vi "InitDeviceAD_8532.vi"(7 "error in (no error)":errorcluster, 10 "task":T1={"Task Info"={"Accele Task"=[], "Simulate"=FALSE, "采样率"={"AISampleRate"=10123, "CouplingType"=10000, "Butter"=1000}, "Trig"={"PreTrigCNT"=0, "TriggerMode"=enum."中间触发", "TriggerSource"=enum."软件触发", "ATRTriggerChannel"=enum."通道0", "TriggerDir"=enum."下降沿触发", "TrigLevelVolt"=0.0, "bAvailableTrig"=FALSE}, "clock"={"EN"=FALSE, "clocksource"=enum."内部时钟", "outclocksource"=enum."Trig0"}, "delay(S)"=0.0}, "datain"={"nSegmentCount"=0, "chaneldataSize"=8192, "t0 in"=timestamp(0 s since 1904-01-01), "nsegmentsize"=0, "chanelcouter"=0}, "times"=0.0, "timer"=[], "\nen"=FALSE} {"Task Info"."采样率"."CouplingType" items=["直流耦合", "交流耦合"]}) -> (0 "error out":errorcluster, 2 "ADBuffer":u16[](array[numeric]), 3 "task out":T1={"Task Info"={"Accele Task"=[], "Simulate"=FALSE, "采样率"={"AISampleRate"=10123, "CouplingType"=10000, "Butter"=1000}, "Trig"={"PreTrigCNT"=0, "TriggerMode"=enum."中间触发", "TriggerSource"=enum."软件触发", "ATRTriggerChannel"=enum."通道0", "TriggerDir"=enum."下降沿触发", "TrigLevelVolt"=0.0, "bAvailableTrig"=FALSE}, "clock"={"EN"=FALSE, "clocksource"=enum."内部时钟", "outclocksource"=enum."Trig0"}, "delay(S)"=0.0}, "datain"={"nSegmentCount"=0, "chaneldataSize"=8192, "t0 in"=timestamp(0 s since 1904-01-01), "nsegmentsize"=0, "chanelcouter"=0}, "times"=0.0, "timer"=[], "\nen"=FALSE} {"Task Info"."采样率"."CouplingType" items=["直流耦合", "交流耦合"]})   [LabVIEW 2009]
uses:
  Data.vi
  PCI8532_32.dll
  Ctrls/Acceleration Channel Config_Ctrls-某型振动实验台测试系统.ctl
  Ctrls/Sample Information.ctl
  Ctrls/Trig.ctl
  Ctrls/clock.ctl
  Ctrls/Task Info.ctl
  Ctrls/task.ctl
  Ctrls/DATA info.ctl
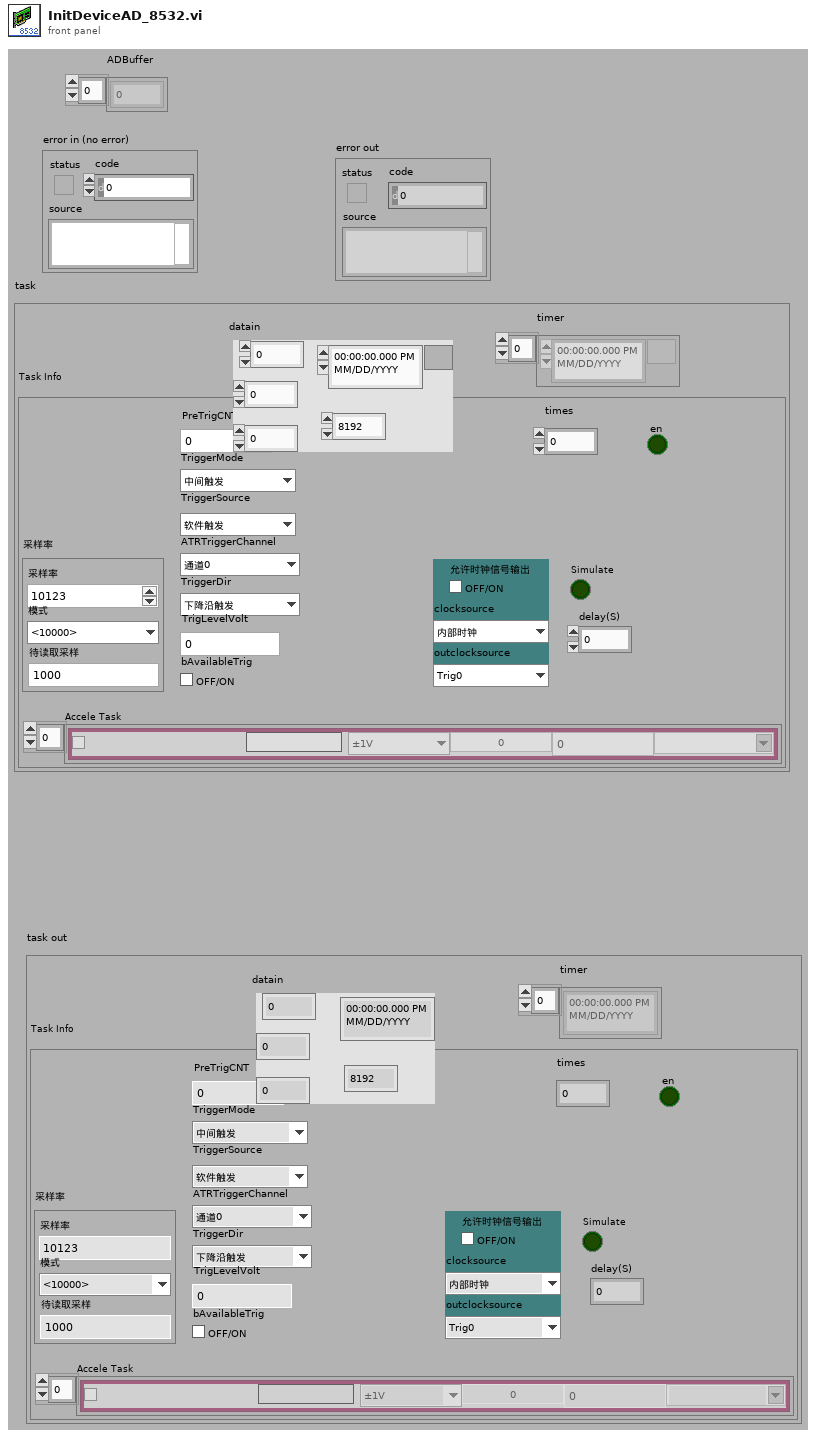
[diagram p1: front panel]
types:
  T1 = typedef "task.ctl" = cluster{"Task Info":T2, "datain":T7, "times":dbl, "timer":timestamp[], "\nen":bool}
  T2 = typedef "Task Info.ctl" = cluster{"Accele Task":T3[], "Simulate":bool, "采样率":T4, "Trig":T5, "clock":T6, "delay(S)":dbl}
  T3 = typedef "Acceleration Channel Config_Ctrls-某型振动实验台测试系统.ctl" = cluster{"Enable":bool, "Name":string, "range":enum16{"±1V", "±5V"}, "SensValue":dbl, "PhysicalName":string, "off":dbl, "Sensunits":string}
  T4 = typedef "Sample Information.ctl" = cluster{"AISampleRate":i32, "CouplingType":i32, "Butter":i32}
  T5 = typedef "Trig.ctl" = cluster{"PreTrigCNT":i32, "TriggerMode":enum16{"中间触发", "后触发", "预触发", "硬件延时触发"}, "TriggerSource":enum16{"软件触发", "DTR信号源", "ATR信号源", "Triger信号触发"}, "ATRTriggerChannel":enum16{"通道0", "通道1", "通道2", "通道3"}, "TriggerDir":enum16{"下降沿触发", "上升沿触发", "上下边没均触发"}, "TrigLevelVolt":sgl, "bAvailableTrig":bool}
  T6 = typedef "clock.ctl" = cluster{"EN":bool, "clocksource":enum16{"内部时钟", "外部时钟"}, "outclocksource":enum16{"Trig0", "Trig1", "Trig2", "Trig3", "Trig4", "Trig5", "Trig6", "Trig7", "PXI_STAR"}}
  T7 = typedef "DATA info.ctl" = cluster{"nSegmentCount":i32, "chaneldataSize":i32, "t0 in":timestamp, "nsegmentsize":i32, "chanelcouter":i32}
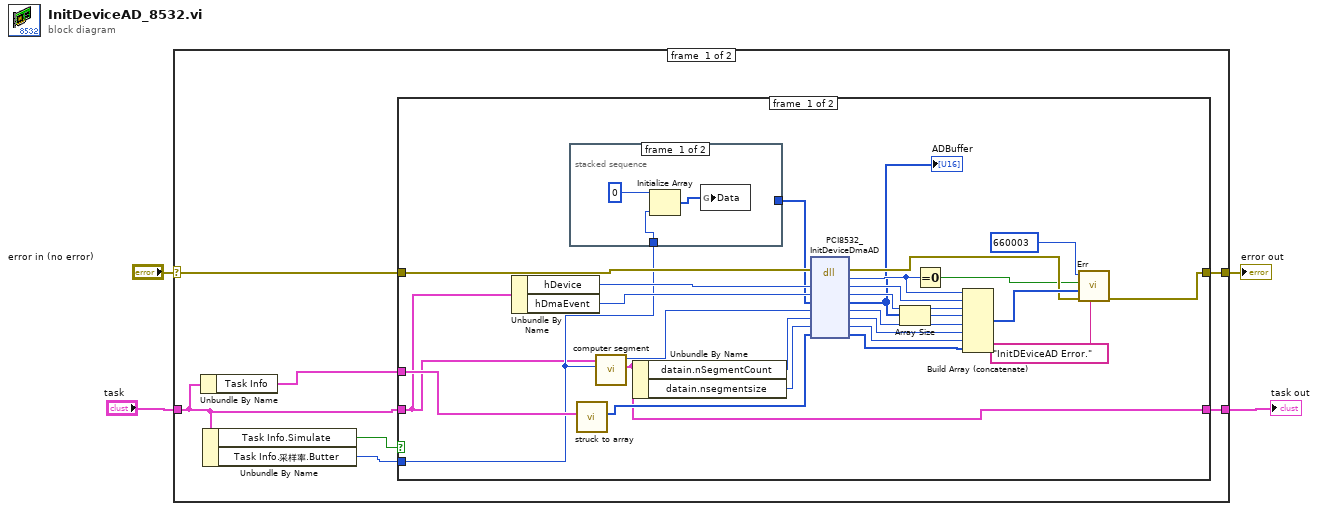
[diagram p0: block diagram]
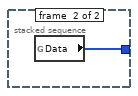
[diagram p2: hidden frame]
diagram:
  n1 = case shown="无错误" "error in (no error)" {
    selector: "error in (no error)" -> [w9 w46]
    tunnel: [w11 w46] -> w4
    tunnel: "task" -> [w8 w45]
    tunnel: [w7 w45] -> w1
    frame #0 {
      n2 = Unbundle By Name(w8) -> ("Task Info"=w6:T2)
      n3 = Unbundle By Name(w8) -> ("Task Info.Simulate"=w10:bool, "Task Info.采样率.Butter"=w5:i32)
      n4 = case shown="假" w10 {
        tunnel: [w36 w44] -> w11
        tunnel: w6 -> [w37 _]
        tunnel: w9 -> [w38 w44]
        tunnel: w5 -> [w16 _]
        tunnel: w8 -> [w15 w43]
        tunnel: [w12 w43] -> w7
        frame #0 {
          n5 = Unbundle By Name(w15) -> ("hDevice"=w24:i32, "hDmaEvent"=w23:i32)
          n6 = stacked-sequence {
            tunnel: [_ w42] -> w17
            tunnel: w16 -> [w40 _]
            frame #0 {
              n7 = Initialize Array(u16 0, w40) -> (w39:u16[])
              n8 = global write "Data.vi" "Data"(w39) -> ()
            }
            frame #1 {
              n9 = global read "Data.vi" "Data"() -> (w42:u16[])
            }
          }
          n10 = call "struck to array.vi"("Task Info"=w37) -> ("array"=w25:i32[])  [unwired: 10 out]
          n11 = call "computer segment.vi"("Buffer"=w16, "task"=w15) -> ("output cluster"=w12:T1, "nReadsizeword"=w22:i32)  [unwired: 8 out]
          n12 = Unbundle By Name(w12) -> ("datain.nSegmentCount"=w14:i32, "datain.nsegmentsize"=w13:i32)
          n13 = dll-call lib="PCI8532_32.dll" fn="PCI8532_InitDeviceDmaAD" label="InitDeviceDmaAD"(error in=w38, "hDevice"=w24, "hDmaEvent"=w23, "ADBuffer"=w17, "nReadSizeWords"=w22, "nSegmentCount"=w14, "nSegmentSizeWords"=w13, "pAPara"=w25) -> (error out=w21:errorcluster, "返回类型"=w33:i32, "hDevice"=w32:i32, "hDmaEvent"=w31:i32, "ADBuffer"=w18:u16[], "nReadSizeWords"=w30:i32, "nSegmentCount"=w29:i32, "nSegmentSizeWords"=w28:i32, "pAPara"=w27:i32[])  [unwired: 2 in, 1 out]
          "ADBuffer" <- w18
          n14 = Array Size(array=w18) -> (size(s)=w19:i32)
          n15 = Equal To 0?(x=w33) -> (x = 0?=w20:bool)
          n16 = Build Array (concatenate)(w33, w32, w31, w19, w30, w29, w28, w27) -> (w26:i32[])
          n17 = call "Err.vi"("source"="InitDEviceAD Error.", "error in (no error)"=w21, "Par"=w26, "error?"=w20, "code"=660003) -> ("error out"=w36:errorcluster)  [unwired: 6 out]
        }
        frame #1 {
        }
      }
    }
    frame #1 {
    }
  }
  "error out" <- w4
  "task out" <- w1
